vi "measurement computing.vi"() -> ()   [LabVIEW 2012]
panel:
  out "data":dbl[](array[numeric])
  in  "TCs 1-8":u16(ring) items=["Dev0", "Dev1", "Dev2", "Dev3", "Dev4", "Dev5", "Dev6", "Dev7"]
  in  "TCs 9-16":u16(ring)=1 items=["Dev0", "Dev1", "Dev2", "Dev3", "Dev4", "Dev5", "Dev6", "Dev7"]
  in  "stop":bool
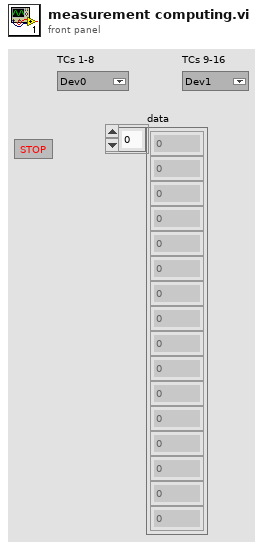
[diagram p1: front panel]
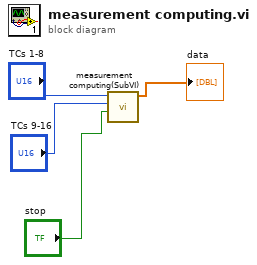
[diagram p0: block diagram]
diagram:
  n1 = call "measurement computing(SubVI).vi"("stop"="stop", "TCs 9-16"="TCs 9-16", "TCs 1-8"="TCs 1-8") -> ("data"=→"data":dbl[])  [unwired: 8 in]
